vi "ttm_logging_poller.vi"() -> ()   [LabVIEW 2011]
uses:
  <vilib>/Utility/file.llb/Write To Spreadsheet File (DBL).vi
panel:
  out "Measurement is going on":bool
  out "Logging is on":bool
  out "Ramp":bool
  out "Cyclic":bool
  out "FullScaleCha3":dbl
  out "FullScaleCha2":dbl
  out "FullScaleCha1":dbl
  out "path":path
  in  "Column Types":i32[][](array[ring])=[[0, 0, 0, 0, 0, 0, 0, 0]] items=["Feedback", "Direct Auxilary"]
  in  "Number of Columns":i32[](array[numeric])=[3]
  in  "Column Channels":i32[][](array[ring])=[[1, 2, 3, 0, 0, 0, 0, 0]] items=["Not Used", "Channel 1/Logging time", "Channel 2/Controlling command", "Channel 3/Controlling error", "Channel 4/Elapsed quarter-cycle counter", "Total accumulated quarter-cycle counter", "Elapsed segment counter", "Total accumulated segment counter", "Servovalve drive", "Block count", "Uncompensated servovalve drive", "Geometric compensation output 1", "Geometric compensation output 2", "Re-Sampling Filter 1", "Re-Sampling Filter 2", "Re-Sampling Filter 3", "Re-Sampling Filter 4", "Outer cascaded controller output", "Delta_P or acceleration compensation (Raw)", "Auxiliary input from the front of the IAC", "Waveform identifier", "Reserved", "Digital I/O and sample playback actions", "Reserved", "Motor current (EIB only)", "Motor instantaneous power (EIB only)", "Motot filtered power (EIB only)", "Motor speed (EIB only)", "Motor viscous loss (EIB only)"]
  in  "Interval/Buffer Parameters":T1={"Sample interval - ms (2)"=2.0, "Buffer Length (1000)"=100, "No. of Buffers (0)"=0} {"Sample interval - ms (2)" min=0.2 format="%.1f"}
  out "Waveform Graph 2":dbl[][](graph)
  # "datalogger internal \npreferences:"
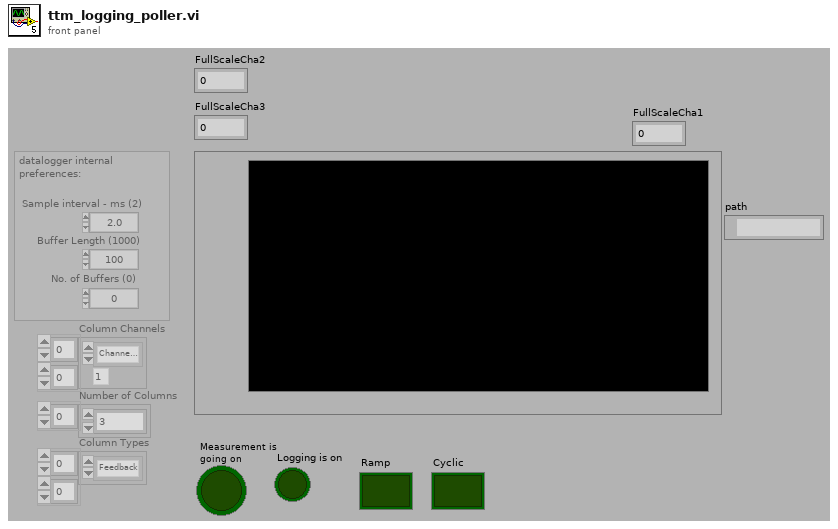
[diagram p1: front panel]
types:
  T1 = cluster{"Sample interval - ms (2)":dbl, "Buffer Length (1000)":i32, "No. of Buffers (0)":i32}
  T2 = cluster{"Name":string, "Type":i32, "SI Full Scale":dbl, "Full Scale":dbl, "Units String":string, "Display Format":string, "Gauge Length":dbl}[][]
  T3 = cluster{"Device ID":i32, "Device Name":string, "Device Type":i32}[]
  T4 = cluster{"Conversion Factors[0]":dbl, "Conversion Factors[1]":dbl, "Conversion Factors[2]":dbl, "Conversion Factors[3]":dbl, "Conversion Factors[4]":dbl, "Conversion Factors[5]":dbl, "Conversion Factors[6]":dbl, "Conversion Factors[7]":dbl, "Conversion Factors[8]":dbl}
  T5 = typedef "NI_Matrix.lvlib/RealMatrix.ctl" = dbl[][]
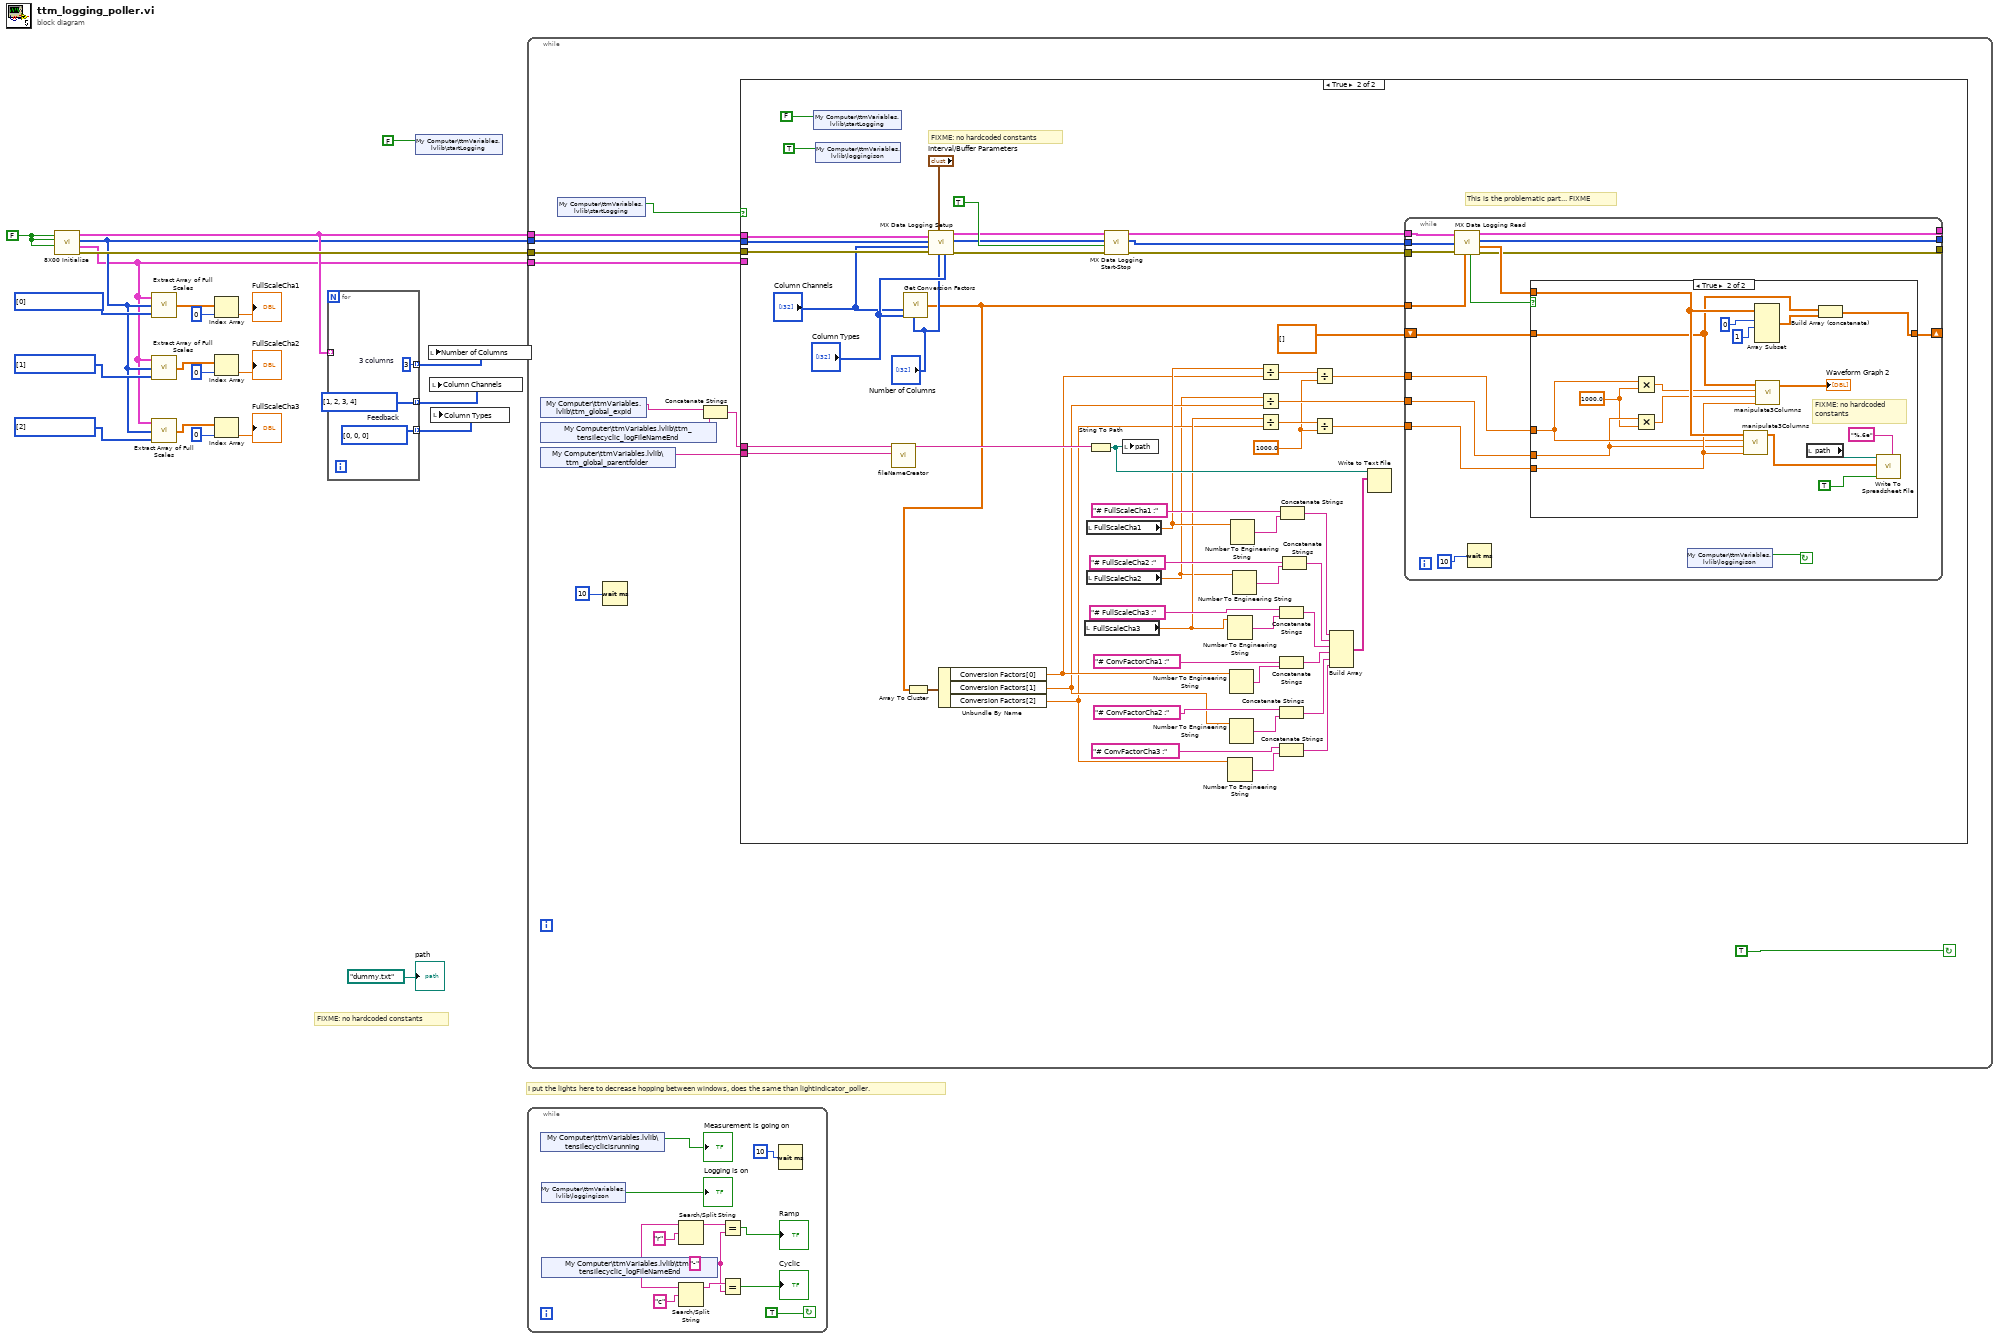
[diagram p0: block diagram]
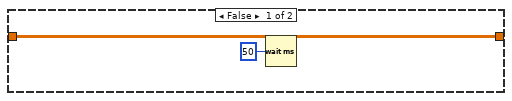
[diagram p3: hidden frame]
diagram:
  w12 = u16[] [2] items=["Channel 1", "Channel 2", "Channel 3", "Channel 4"] ("Channel")
  w13 = u16[] [1] items=["Channel 1", "Channel 2", "Channel 3", "Channel 4"] ("Channel")
  w15 = u16[] [0] items=["Channel 1", "Channel 2", "Channel 3", "Channel 4"] ("Channel")
  w22 = FALSE ("Create Console? (T)")
  # "I put the lights here to decrease hopping between windows, does the same than lightIndicator_poller."
  # "FIXME: no hardcoded constants"
  n1 = call "8X00 Initialise.vi"("Reset?"=w22, "Create DVM? (T)"=w22, "Create Console? (T)"=w22) -> ("error out"=w21:errorcluster, "Channel Data"=w1:T2, "Axis Selector"=w11:i32[], "Axis Information"=w16:T3)  [unwired: 1 in]
  n2 = call "Extract Array of Full Scales.vi"("Channel"=w15, "Axis Selector"=w11, "Axis\nChannel"=w1) -> ("Full Scales"=w10:dbl[])
  n3 = call "Extract Array of Full Scales.vi"("Channel"=w13, "Axis Selector"=w11, "Axis\nChannel"=w1) -> ("Full Scales"=w2:dbl[])
  n4 = call "Extract Array of Full Scales.vi"("Channel"=w12, "Axis Selector"=w11, "Axis\nChannel"=w1) -> ("Full Scales"=w3:dbl[])
  n5 = Index Array(array=w10, index=0) -> (element=→"FullScaleCha1":dbl)
  n6 = Index Array(array=w2, index=0) -> (element=→"FullScaleCha2":dbl)
  n7 = Index Array(array=w3, index=0) -> (element=→"FullScaleCha3":dbl)
  n8 = for {
    tunnel: [w25] -> w19 mode=indexing
    tunnel: [w24] -> w17 mode=indexing
    tunnel: [3] -> w18 mode=indexing
    tunnel: w16 -> [_] mode=indexing
    w24 = i32[] [0, 0, 0]  # Feedback
    w25 = i32[] [1, 2, 3, 4]  # 3 columns
  }
  n9 = shared-variable "My Computer\\ttmVariables.lvlib\\startLogging"(FALSE ("startLogging")) -> ()  [unwired: 1 in, 1 out]
  n10 = local write "Number of Columns"(w18) -> ()
  n11 = local write "Column Channels"(w19) -> ()
  n12 = local write "Column Types"(w17) -> ()
  n13 = while {
    tunnel: w16 -> [w34]
    tunnel: w11 -> [w33]
    tunnel: w21 -> [w32]
    tunnel: w1 -> [w30]
    stop <- TRUE continue-if-true
    n14 = shared-variable "My Computer\\ttmVariables.lvlib\\ttm_global_expid"() -> (w26:string)  [unwired: 1 in, 1 out]
    n15 = shared-variable "My Computer\\ttmVariables.lvlib\\ttm_tensilecyclic_logFileNameEnd"() -> (w28:string)  [unwired: 1 in, 1 out]
    n16 = shared-variable "My Computer\\ttmVariables.lvlib\\ttm_global_parentfolder"() -> (w29:string)  [unwired: 1 in, 1 out]
    n17 = shared-variable "My Computer\\ttmVariables.lvlib\\startLogging"() -> (w31:bool)  [unwired: 1 in, 1 out]
    n18 = Wait (ms)(milliseconds to wait=u32 10) -> ()  [unwired: 1 out]
    n19 = Concatenate Strings(w26, w28) -> (w27:string)
    n20 = case shown="True" w31 {
      tunnel: w34 -> [_ w81]
      tunnel: w33 -> [_ w82]
      tunnel: w32 -> [_ w83]
      tunnel: w27 -> [_ w41]
      tunnel: w30 -> [_ _]
      tunnel: w29 -> [_ w43]
      frame False {
      }
      frame True {
        w38 = 1000.0 ("y")
        # "FIXME: no hardcoded constants"
        # "This is the problematic part... FIXME"
        n21 = shared-variable "My Computer\\ttmVariables.lvlib\\startLogging"(FALSE ("startLogging")) -> ()  [unwired: 1 in, 1 out]
        n22 = shared-variable "My Computer\\ttmVariables.lvlib\\loggingison"(TRUE ("loggingison")) -> ()  [unwired: 1 in, 1 out]
        n23 = call "fileNameCreator.vi"("folder"=w43, "Measurement ID"=w41) -> ("concatenated string"=w75:string)  [unwired: 9 in]
        n24 = call "Get Conversion Factors.vi"("Column Channels"="Column Channels", "Column Types"="Column Types", "Number of Columns"="Number of Columns") -> ("Conversion Factors"=w63:dbl[])  [unwired: 2 in]
        n25 = Array To Cluster(array=w63) -> (cluster=w37:T4)
        n26 = call "MX Data Logging Setup.vi"("Column Types"="Column Types", "Number of Columns"="Number of Columns", "Interval/Buffer Parameters"="Interval/Buffer Parameters", "error in (no error)"=w83, "Column Channels"="Column Channels", "Axis Selector"=w82, "Axis Information"=w81) -> ("error out"=w87:errorcluster, "Axis Selector copy"=w77:i32[], "Axis Information out"=w78:T3)  [unwired: 1 out]
        n27 = Unbundle By Name(w37) -> ("Conversion Factors[0]"=w52:dbl, "Conversion Factors[1]"=w51:dbl, "Conversion Factors[2]"=w48:dbl)
        n28 = local read "FullScaleCha3"() -> (w49:dbl)
        n29 = local read "FullScaleCha1"() -> (w53:dbl)
        n30 = local read "FullScaleCha2"() -> (w39:dbl)
        n31 = String To Path(string=w75) -> (path=w74:path)
        n32 = call "MX Data Logging Start-Stop.vi"("error in (no error)"=w87, "Start (T)"=TRUE, "Axis Selector"=w77, "Axis Information"=w78) -> ("error out"=w84:errorcluster, "Axis Selector copy"=w85:i32[], "Axis Information out"=w86:T3)  [unwired: 4 in]
        n33 = local write "path"(w74) -> ()
        n34 = Number To Engineering String(4:w49) -> (0:w64:string)  [unwired: 3 in]
        n35 = Number To Engineering String(4:w48) -> (0:w55:string)  [unwired: 3 in]
        n36 = Number To Engineering String(4:w52) -> (0:w61:string)  [unwired: 3 in]
        n37 = Number To Engineering String(4:w51) -> (0:w58:string)  [unwired: 3 in]
        n38 = Number To Engineering String(4:w53) -> (0:w70:string)  [unwired: 3 in]
        n39 = Number To Engineering String(4:w39) -> (0:w68:string)  [unwired: 3 in]
        n40 = Divide(x=w53, y=w52) -> (x/y=w47:dbl)
        n41 = Divide(x=w39, y=w51) -> (x/y=w50:dbl)
        n42 = Divide(x=w49, y=w48) -> (x/y=w46:dbl)
        n43 = Concatenate Strings("# FullScaleCha3 :", w64) -> (w65:string)
        n44 = Concatenate Strings("# ConvFactorCha1 :", w61) -> (w60:string)
        n45 = Concatenate Strings("# ConvFactorCha2 :", w58) -> (w57:string)
        n46 = Concatenate Strings("# ConvFactorCha3 :", w55) -> (w54:string)
        n47 = Concatenate Strings("# FullScaleCha1 :", w70) -> (w72:string)
        n48 = Concatenate Strings("# FullScaleCha2 :", w68) -> (w67:string)
        n49 = Divide(x=w47, y=w38) -> (x/y=w40:dbl)
        n50 = Divide(x=w46, y=w38) -> (x/y=w45:dbl)
        n51 = Build Array(w72, w67, w65, w60, w57, w54) -> (w73:string[])
        n52 = Write to Text File(file (use dialog)=w74, text=w73) -> ()  [unwired: 2 in, 3 out]
        n53 = while {
          tunnel: [w98] -> _
          tunnel: [w99] -> _
          tunnel: w84 -> [w102]
          tunnel: w63 -> [w101]
          tunnel: w85 -> [w103]
          tunnel: w86 -> [w104]
          tunnel: [w97] -> _
          shift-right: [w96] -> _
          shift-left: dbl[][] [] -> [w95]
          tunnel: w40 -> [w93]
          tunnel: w50 -> [w92]
          tunnel: w45 -> [w91]
          stop <- w94 continue-if-true
          n54 = call "MX Data Logging Read.vi"("Axis Information"=w104, "Axis Selector"=w103, "error in (no error)"=w102, "Conversion Values (100)"=w101) -> ("Axis Information copy"=w97:T3, "Axis Selector copy"=w99:i32[], "Data Available"=w100:bool, "Collected Data - Eng Units"=w105:dbl[][], "error out"=w98:errorcluster)  [unwired: 2 out]
          n55 = Wait (ms)(milliseconds to wait=u32 10) -> ()  [unwired: 1 out]
          n56 = case shown="True" w100 {
            tunnel: w105 -> [_ w118]
            tunnel: [w107 w122] -> w96
            tunnel: w95 -> [w107 w109]
            tunnel: w93 -> [_ w115]
            tunnel: w92 -> [_ w113]
            tunnel: w91 -> [_ w116]
            frame False {
              n57 = Wait (ms)(milliseconds to wait=u32 50) -> ()  [unwired: 1 out]
            }
            frame True {
              w112 = 1000.0 ("y")
              # "FIXME: no hardcoded \nconstants"
              n58 = Multiply(x=w115, y=w112) -> (x*y=w114:dbl)
              n59 = Multiply(x=w113, y=w112) -> (x*y=w111:dbl)
              n60 = call "manipulate3Columns.vi"("Col2Mul"=w116, "Col1Mul"=w113, "Col0Mul"=w115, "Real Matrix"=w118) -> ("submatrix"=w117:T5)  [unwired: 7 in]
              n61 = Array Subset(array=w118, index (row)=0 ("index"), length (row)=1 ("length")) -> (w123:dbl[][])  [unwired: 2 in]
              n62 = call "manipulate3Columns.vi"("Col2Mul"=w116, "Col1Mul"=w111, "Col0Mul"=w114, "Real Matrix"=w109) -> ("submatrix"=→"Waveform Graph 2":T5)  [unwired: 7 in]
              n63 = local read "path"() -> (w119:path)
              n64 = Build Array (concatenate)(w109, w123) -> (w122:dbl[][])
              n65 = call-poly <vilib>:"Write To Spreadsheet File.vi"("format (%.3f)"="%.6e", "append to file? (new file:F)"=TRUE, "2D data"=w117, "file path (dialog if empty)"=w119) -> ()  [unwired: 4 in, 1 out]
            }
          }
          n66 = shared-variable "My Computer\\ttmVariables.lvlib\\loggingison"() -> (w94:bool)  [unwired: 1 in, 1 out]
        }
      }
    }
  }
  n67 = while {
    stop <- TRUE continue-if-true
    w132 = "-"
    n68 = shared-variable "My Computer\\ttmVariables.lvlib\\tensilecyclicisrunning"() -> (→"Measurement is going on":bool)  [unwired: 1 in, 1 out]
    n69 = shared-variable "My Computer\\ttmVariables.lvlib\\loggingison"() -> (→"Logging is on":bool)  [unwired: 1 in, 1 out]
    n70 = shared-variable "My Computer\\ttmVariables.lvlib\\ttm_tensilecyclic_logFileNameEnd"() -> (w131:string)  [unwired: 1 in, 1 out]
    n71 = Search/Split String(string=w131, search string/char (-)="r") -> (substring before match=w133:string)  [unwired: 1 in, 2 out]
    n72 = Search/Split String(string=w131, search string/char (-)="c") -> (substring before match=w134:string)  [unwired: 1 in, 2 out]
    n73 = Equal?(x=w133, y=w132) -> (x = y?=→"Ramp":bool)
    n74 = Equal?(x=w134, y=w132) -> (x = y?=→"Cyclic":bool)
    n75 = Wait (ms)(milliseconds to wait=u32 10) -> ()  [unwired: 1 out]
  }
  "path" <- path "dummy.txt" ("path")
